vi "Bitfile Component Check.vi"(2 "error in (no error)":errorcluster, 3 "Control Scalars":T2) -> (0 "error out":errorcluster, 1 "Valid?":bool)   [LabVIEW 2011, in "Sensor Simulation Custom Device.lvlib"]
uses:
  Sensor Simulation Custom Device.lvlib
  <userlib>/_FPGA Interface Advanced Tools/FPGA Bitfile Utility/TypeDefs/Scalar Register Set.ctl
  <userlib>/_FPGA Interface Advanced Tools/FPGA Bitfile Utility/TypeDefs/Scalar Register.ctl
  TypeDefs/xVDT.ctl
  <userlib>/_FPGA Interface Advanced Tools/FPGA Bitfile Utility/FPGA Bitfile Utility.lvlib
panel:
  out "xVDTs":T1[](array[typedef])
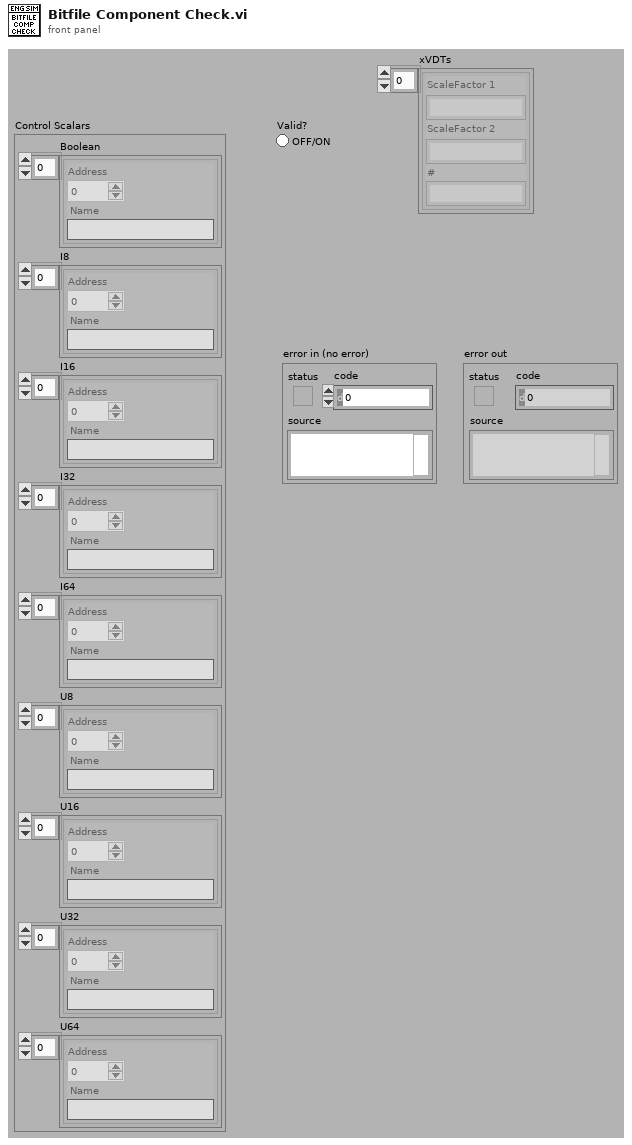
[diagram p1: front panel]
types:
  T1 = typedef "Sensor Simulation Custom Device.lvlib/xVDT.ctl" = cluster{"ScaleFactor 1":string, "ScaleFactor 2":string, "#":string}
  T2 = typedef "FPGA Bitfile Utility.lvlib/Scalar Register Set.ctl" = cluster{"Boolean":T3[], "I8":T3[], "I16":T3[], "I32":T3[], "I64":T3[], "U8":T3[], "U16":T3[], "U32":T3[], "U64":T3[]}
  T3 = typedef "FPGA Bitfile Utility.lvlib/Scalar Register.ctl" = cluster{"Address":u32, "Name":string}
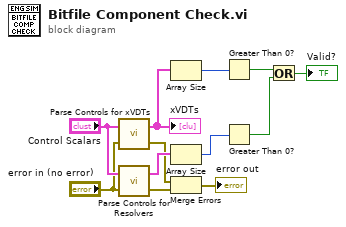
[diagram p0: block diagram]
diagram:
  n1 = call "Parse Controls for xVDTs.vi"("error in (no error)"="error in (no error)", "Control Scalars"="Control Scalars") -> ("error out"=w3:errorcluster, "xVDTs"=w12:T1[])
  "xVDTs" <- w12
  n2 = call "Parse Controls for Resolvers.vi"("error in (no error)"="error in (no error)", "Control Scalars"="Control Scalars") -> ("error out"=w2:errorcluster, "Resolvers"=w7:T1[])
  n3 = Array Size(array=w12) -> (size(s)=w11:i32)
  n4 = Array Size(array=w7) -> (size(s)=w8:i32)
  n5 = Merge Errors(w3, w2) -> (→"error out":errorcluster)
  n6 = Greater Than 0?(x=w11) -> (x > 0?=w10:bool)
  n7 = Greater Than 0?(x=w8) -> (x > 0?=w5:bool)
  n8 = Or(x=w10, y=w5) -> (x .or. y?=→"Valid?":bool)
